vi "dfd_Matched ZP Pair to SOS.vi"(10 "gain":dbl=1.0, 11 "Matched ZP Pair":cluster{"zeros":cdb[], "poles":cdb[]}[](array[cluster])) -> (2 "SOS reverse coefficients":dbl[](array[numeric]), 3 "SOS forward coefficients":dbl[](array[numeric]))   [LabVIEW 2017, in "NI_DigFilterLicensed.lvlib"]
uses:
  <vilib>/addons/Digital Filter Design/NI_DigFilterLicensed.lvlib
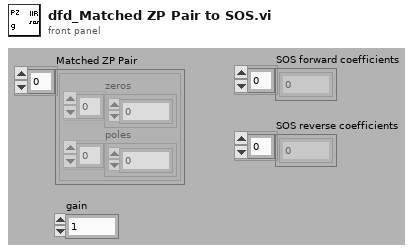
[diagram p1: front panel]
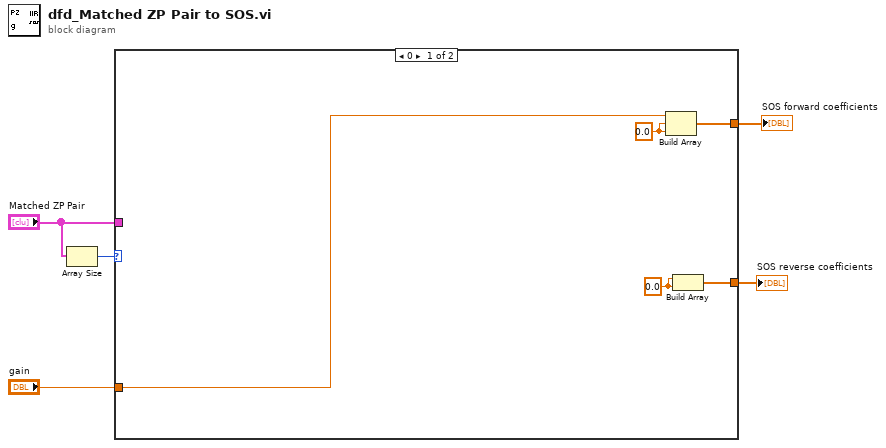
[diagram p0: block diagram]
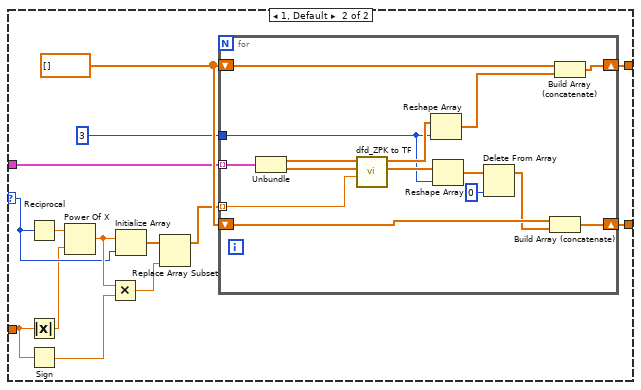
[diagram p2: hidden frame]
diagram:
  n1 = Array Size(array="Matched ZP Pair") -> (size(s)=w2:i32)
  n2 = case shown="0" w2 {
    selector: w2 -> [_ w14]
    tunnel: [w10 w24] -> w5
    tunnel: [w8 w23] -> w4
    tunnel: "Matched ZP Pair" -> [_ w20]
    tunnel: "gain" -> [w9 w13]
    frame 0 {
      w7 = 0.0 ("element")
      w6 = 0.0 ("element")
      n3 = Build Array(w9, w7, w7) -> (w8:dbl[])
      n4 = Build Array(w6, w6) -> (w10:dbl[])
    }
    frame 1, Default {
      w22 = dbl[] []
      n5 = Reciprocal(x=w14) -> (1/x=w19:dbl)
      n6 = Absolute Value(x=w13) -> (abs(x)=w12:dbl)
      n7 = Sign(1:w13) -> (0:w11:dbl)
      n8 = Power Of X(1:w12, 2:w19) -> (0:w17:dbl)
      n9 = Multiply(x=w17, y=w11) -> (x*y=w16:dbl)
      n10 = Initialize Array(w17, w14) -> (w18:dbl[])
      n11 = Replace Array Subset(array=w18, new element=w16) -> (w15:dbl[])  [unwired: 1 in]
      n12 = for {
        tunnel: w20 -> [w39] mode=indexing
        shift-right: [w38] -> w23
        shift-left: w22 -> [w37]
        shift-right: [w35] -> w24
        shift-left: w22 -> [w36]
        tunnel: 3 ("dimension size") -> [w29]
        tunnel: w15 -> [w25] mode=indexing
        n13 = Unbundle(w39) -> ("zeros"=w34:cdb[], "poles"=w33:cdb[])
        n14 = call <vilib>:"dfd_ZPK to TF.vi"("gain"=w25, "poles"=w33, "zeros"=w34) -> ("denominator"=w30:dbl[], "numerator"=w32:dbl[])  [unwired: 7 out]
        n15 = Reshape Array(w32, w29) -> (w31:dbl[])
        n16 = Reshape Array(w30, w29) -> (w28:dbl[])
        n17 = Delete From Array(array=w28, index=0) -> (array with subset deleted=w26:dbl[])  [unwired: 1 in, 1 out]
        n18 = Build Array (concatenate)(w36, w26) -> (w35:dbl[])
        n19 = Build Array (concatenate)(w37, w31) -> (w38:dbl[])
      }
    }
  }
  "SOS reverse coefficients" <- w5
  "SOS forward coefficients" <- w4
